vi "Write Color.vi"(8 "error in (no error)":errorcluster, 10 "Color":T1[](array[typedef]), 11 "Flags in":refnum<class "Flags.lvclass">) -> (0 "error out":errorcluster, 3 "Flags out":refnum<class "Flags.lvclass">)   [LabVIEW 2015, in "Flags.lvclass"]
uses:
  Flags.lvclass
  ColorEnum.ctl
  Flags.lvclass/Flags.ctl
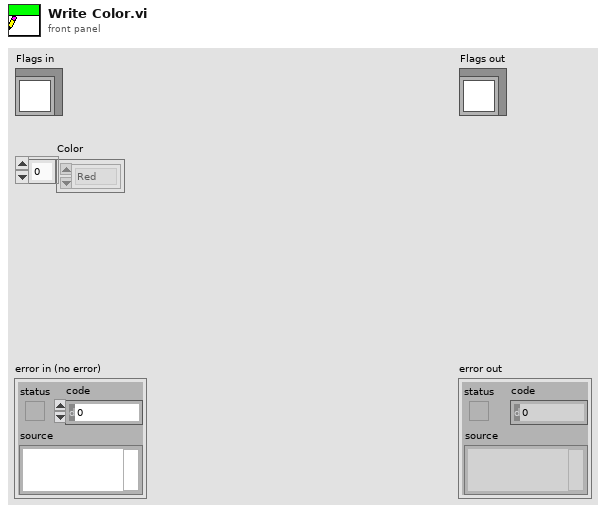
[diagram p1: front panel]
types:
  T1 = typedef "Flags.lvclass/ColorEnum.ctl" = enum8{"Red", "Blue", "Green", "Yellow"}
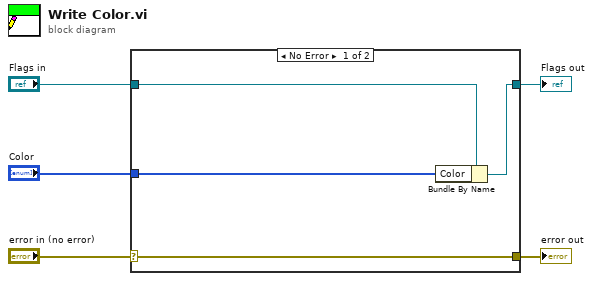
[diagram p0: block diagram]
diagram:
  n1 = case shown="No Error" "error in (no error)" {
    selector: "error in (no error)" -> [w9 w10]
    tunnel: [w9 w10] -> w4
    tunnel: [w7 w11] -> w2
    tunnel: "Flags in" -> [w8 w11]
    tunnel: "Color" -> [w6 _]
    frame No Error {
      n2 = Bundle By Name(cluster=w8, "Color"=w6) -> (w7:refnum<class "Flags.lvclass">)
    }
    frame Error {
    }
  }
  "error out" <- w4
  "Flags out" <- w2
